vi "Q.Dequeue + Error Check.vi"(8 "Error In":errorcluster, 10 "Timeout(-1)":i32=-1, 11 "Q In":refnum<queue>) -> (0 "error out":errorcluster, 2 "Cmd":string, 3 "Q Out":refnum<queue>, 4 "Data1":variant, 5 "Sub":string, 6 "Data2":variant)   [LabVIEW 2024, in "EQMF.lvlib" / "Queue Utils.lvlib"]
uses:
  Queue Utils.lvlib
  Q.Element.ctl
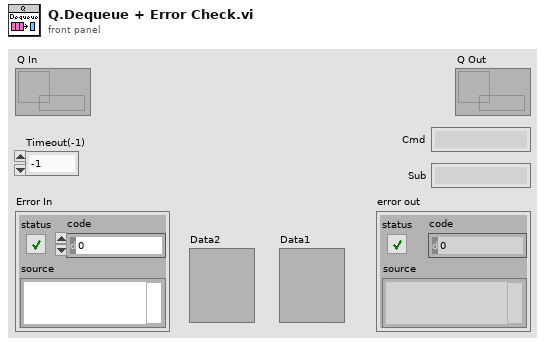
[diagram p1: front panel]
types:
  T1 = typedef "EQMF.lvlib/Queue Utils.lvlib/Q.Element.ctl" = cluster{"Cmd":string, "Sub":string, "Data1":variant, "Data2":variant}
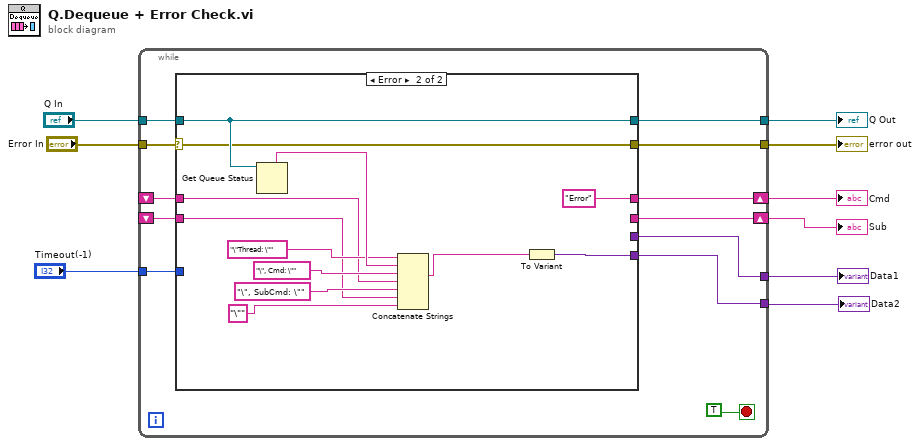
[diagram p0: block diagram]
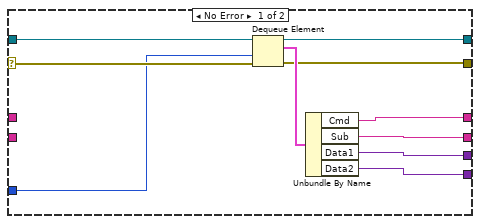
[diagram p2: hidden frame]
diagram:
  n1 = while {
    shift-right: [w16] -> w3
    shift-left: _ -> [w18]
    shift-right: [w15] -> w4
    shift-left: _ -> [w17]
    tunnel: "Q In" -> [w20]
    tunnel: [w12] -> w7
    tunnel: "Error In" -> [w21]
    tunnel: [w11] -> w6
    tunnel: [w14] -> w5
    tunnel: [w13] -> w2
    tunnel: "Timeout(-1)" -> [w10]
    stop <- TRUE stop-if-true
    n2 = case shown="Error" w21 {
      selector: w21 -> [w29 w32]
      tunnel: w20 -> [w30 w39]
      tunnel: [w28 w39] -> w12
      tunnel: [w27 w32] -> w11
      tunnel: w18 -> [_ w38]
      tunnel: w17 -> [_ w37]
      tunnel: [w26 "Error"] -> w16
      tunnel: [w25 _] -> w15
      tunnel: [w24 _] -> w14
      tunnel: [w23 w34] -> w13
      tunnel: w10 -> [w22 _]
      frame No Error {
        n3 = Dequeue Element(queue=w30, timeout in ms (-1)=w22, error in (no error)=w29) -> (queue out=w28:refnum<queue>, element=w31:T1, error out=w27:errorcluster)  [unwired: 1 out]
        n4 = Unbundle By Name(w31) -> ("Cmd"=w26:string, "Sub"=w25:string, "Data1"=w24:variant, "Data2"=w23:variant)
      }
      frame Error {
        n5 = Get Queue Status(queue=w39) -> (queue name=w43:string)  [unwired: 2 in, 7 out]
        n6 = Concatenate Strings("\"Thread: \"", w43, "\", Cmd: \"", w38, "\", SubCmd: \"", w37, "\"") -> (w33:string)
        n7 = To Variant(anything=w33) -> (Variant=w34:variant)
      }
    }
  }
  "Q Out" <- w7
  "error out" <- w6
  "Data1" <- w5
  "Sub" <- w4
  "Cmd" <- w3
  "Data2" <- w2
